vi "table_to_array_POND.vi"(6 "usuario_registra":i32, 8 "error in (no error)":errorcluster, 9 "Tabla Referencia Acústica Generador Externo":string[][](array[string]), 10 "id_pon_frecuencia":i32, 11 "last_id_ajuste_previo":string) -> (0 "error out":errorcluster, 3 "Array":string[](array[string]))   [LabVIEW 2019, in "Base de Datos.lvclass"]
uses:
  Base de Datos.lvclass
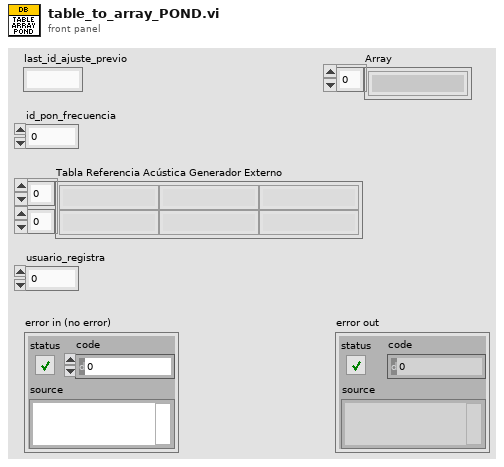
[diagram p1: front panel]
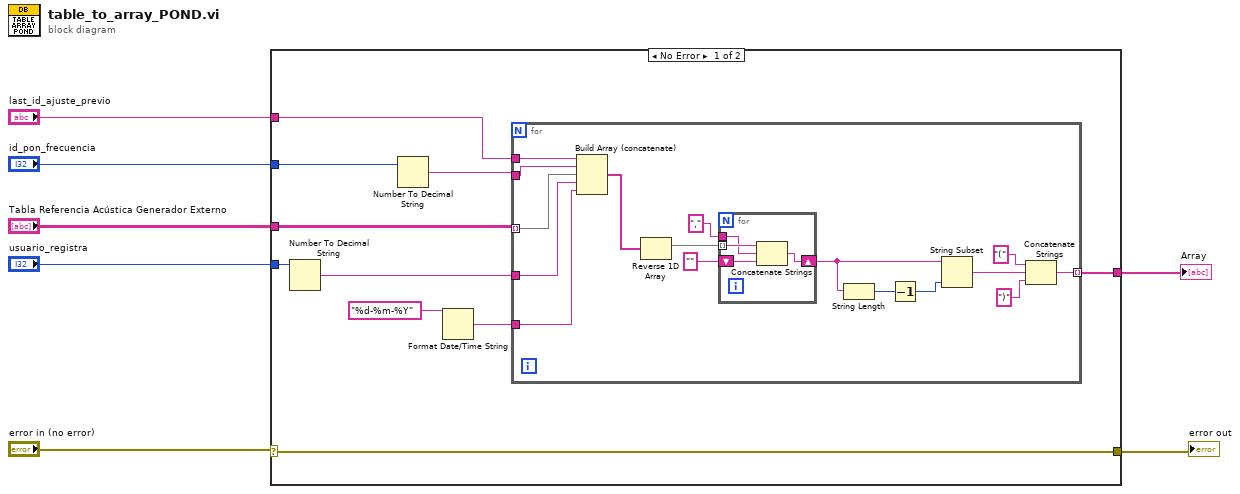
[diagram p0: block diagram]
diagram:
  n1 = case shown="No Error" "error in (no error)" {
    selector: "error in (no error)" -> [w9 w38]
    tunnel: "usuario_registra" -> [w16 _]
    tunnel: "id_pon_frecuencia" -> [w15 _]
    tunnel: [w13 _] -> w5
    tunnel: "Tabla Referencia Acústica Generador Externo" -> [w12 _]
    tunnel: "last_id_ajuste_previo" -> [w8 _]
    tunnel: [w9 w38] -> w1
    frame No Error {
      n2 = Number To Decimal String(number=w16) -> (decimal integer string=w17:string)  [unwired: 1 in]
      n3 = Number To Decimal String(number=w15) -> (decimal integer string=w14:string)  [unwired: 1 in]
      n4 = Format Date/Time String(time format string (%c)="%d-%m-%Y") -> (date/time string=w11:string)  [unwired: 2 in]
      n5 = for {
        tunnel: w14 -> [w33]
        tunnel: w17 -> [w32]
        tunnel: w11 -> [w31]
        tunnel: w12 -> [w24] mode=indexing
        tunnel: [w22] -> w13 mode=indexing
        tunnel: w8 -> [w18]
        n6 = Build Array (concatenate)(w18, w33, w24, w32, w31) -> (w29:string[])
        n7 = Reverse 1D Array(array=w29) -> (reversed array=w28:string[])
        n8 = for {
          shift-right: [w37] -> w27
          shift-left: "" -> [w36]
          tunnel: w28 -> [w35] mode=indexing
          tunnel: "," ("string") -> [w34]
          n9 = Concatenate Strings(w35, w34, w36) -> (w37:string)
        }
        n10 = String Length(string=w27) -> (length=w26:i32)
        n11 = Decrement(x=w26) -> (x-1=w25:i32)
        n12 = String Subset(string=w27, length (rest)=w25) -> (substring=w23:string)  [unwired: 1 in]
        n13 = Concatenate Strings("(" ("element"), w23, ")" ("element")) -> (w22:string)
      }
    }
    frame Error {
    }
  }
  "Array" <- w5
  "error out" <- w1
